vi "Labspec Video.vi"(8 "error in":errorcluster, 9 "Mode":T1 items=["Start Video", "Stop Video", "Get Video ID", "Start Extended Video"], 11 "Automation Refnum In":refnum<k7>) -> (0 "error out":errorcluster, 1 "Video ID":i32, 3 "Automation Refnum Out":refnum<k7>)   [LabVIEW 2014]
uses:
  NGSLabspec/NGSLabSpec.llb/Video Mode.ctl
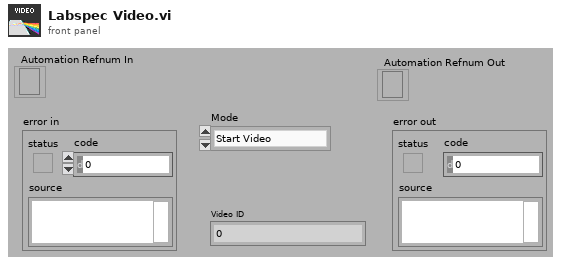
[diagram p1: front panel]
types:
  T1 = typedef "Video Mode.ctl" = u16
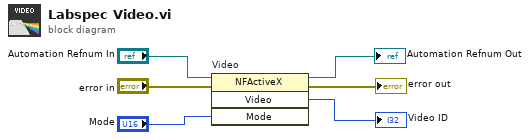
[diagram p0: block diagram]
diagram:
  n1 = invoke on="Video" class="NFActiveX" method="Video"(reference="Automation Refnum In", error in="error in", "Mode"="Mode") -> (reference out=→"Automation Refnum Out":refnum<k7>, error out=→"error out":errorcluster, "Video"=→"Video ID":i32)  [unwired: 1 in, 1 out]
